vi "SetCh.vi"(0 "MagiQmw3 in":refnum<class "MagiQmw3.lvclass">, 2 "ch":i32, 7 "freq":dbl, 9 "atten":dbl, 11 "error in (no error)":errorcluster) -> (4 "MagiQmw3 out":refnum<class "MagiQmw3.lvclass">, 15 "error out":errorcluster)   [LabVIEW 2012, in "MagiQmw3.lvclass"]
uses:
  MagiQmw3.lvclass
  MagiQmw3.lvclass/MagiQmw3.ctl
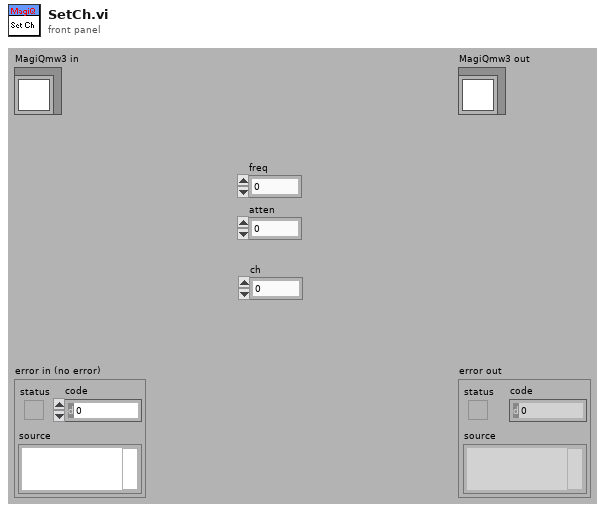
[diagram p1: front panel]
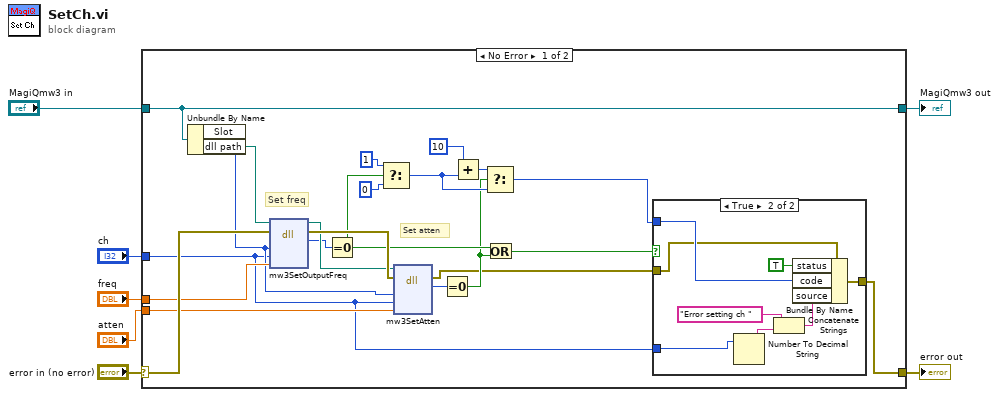
[diagram p0: block diagram]
diagram:
  n1 = case shown="No Error" "error in (no error)" {
    selector: "error in (no error)" -> [w28 w40]
    tunnel: [w9 w40] -> w7
    tunnel: [w29 w39] -> w5
    tunnel: "MagiQmw3 in" -> [w29 w39]
    tunnel: "ch" -> [w12 _]
    tunnel: "freq" -> [w27 _]
    tunnel: "atten" -> [w25 _]
    frame No Error {
      # "Set atten"
      # "Set freq"
      n2 = Unbundle By Name(w29) -> ("Slot"=w13:u16, "dll path"=w23:path)
      n3 = dll-call lib="PulserLib.dll" fn="mw3SetOutputFreq"(path in=w23, error in=w28, "slot"=w13, "ch"=w12, "freq"=w27) -> (path out=w22:path, error out=w26:errorcluster, "return"=w15:i32)  [unwired: 4 in]
      n4 = Equal To 0?(x=w15) -> (x = 0?=w21:bool)
      n5 = Select(t=1, s=w21, f=0) -> (s? t:f=w17:i32)
      n6 = dll-call lib="PulserLib.dll" fn="mw3SetAtten"(path in=w22, error in=w26, "slot"=w13, "ch"=w12, "loss"=w25) -> (error out=w8:errorcluster, "return"=w24:i32)  [unwired: 4 in, 1 out]
      n7 = Equal To 0?(x=w24) -> (x = 0?=w14:bool)
      n8 = Add(x=10, y=w17) -> (x+y=w16:i32)
      n9 = Select(t=w16, s=w14, f=w17) -> (s? t:f=w11:i32)
      n10 = Or(x=w21, y=w14) -> (x .or. y?=w10:bool)
      n11 = case shown="True" w10 {
        tunnel: w12 -> [_ w36]
        tunnel: [w30 w31] -> w9
        tunnel: w11 -> [_ w33]
        tunnel: w8 -> [w30 w32]
        frame False {
        }
        frame True {
          n12 = Number To Decimal String(number=w36) -> (decimal integer string=w35:string)  [unwired: 1 in]
          n13 = Concatenate Strings("Error setting ch " ("source"), w35) -> (w34:string)
          n14 = Bundle By Name(cluster=w32, "status"=TRUE, "code"=w33, "source"=w34) -> (w31:errorcluster)
        }
      }
    }
    frame Error {
    }
  }
  "error out" <- w7
  "MagiQmw3 out" <- w5
